vi "Configure Alarm Delay Com.vi"(0 "VISA resource name":refnum<visa-resource-name>, 5 "Comm Channel (001)":string="001", 7 "Alarm Delay Time":cluster{"Hour":i32, "Min":i32, "Sec":i32}={"Hour"=0, "Min"=0, "Sec"=10} {"Sec" min=0 max=59; "Min" min=0 max=59; "Hour" min=0 max=24}, 11 "error in (no error)":errorcluster) -> (4 "VISA resource name out":refnum<visa-resource-name>, 6 "Comm Channel":string, 15 "error out":errorcluster)   [LabVIEW 2020, in "Yokogawa GX Series.lvlib"]
doc: "Sets the alarm delay of a communication channel.\n\nCommand: SAlmDlyCom"
uses:
  <instrlib>/Yokogawa GX Series/Yokogawa GX Series.lvlib
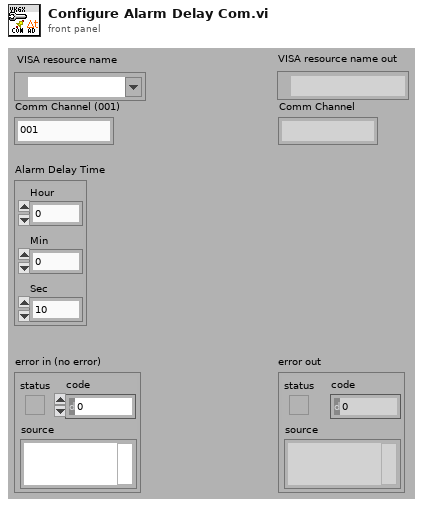
[diagram p1: front panel]
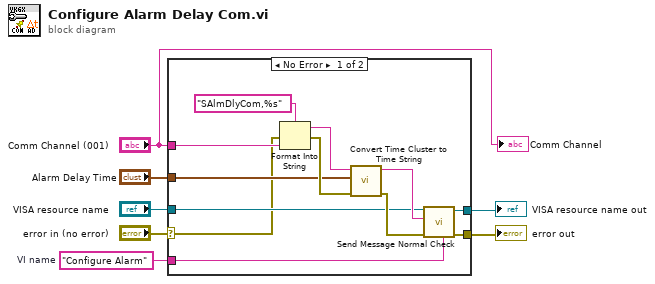
[diagram p0: block diagram]
diagram:
  w3 = "Configure Alarm"  # VI name
  n1 = case shown="No Error" "error in (no error)" {
    selector: "error in (no error)" -> [w8 w20]
    tunnel: [w19 w21] -> w7
    tunnel: "Alarm Delay Time" -> [w13 _]
    tunnel: "VISA resource name" -> [w12 w21]
    tunnel: [w11 w20] -> w4
    tunnel: w3 -> [w10 _]
    tunnel: "Comm Channel (001)" -> [w9 _]
    frame No Error {
      n2 = Format Into String(format string="SAlmDlyCom,%s" ("形式文字列"), error in=w8, w9) -> (resulting string=w17:string, error out=w16:errorcluster)  [unwired: 1 in]
      n3 = call <instrlib>:"Convert Time Cluster to Time String.vi"("error in (no error)"=w16, "Time"=w13, "String"=w17) -> ("error out"=w14:errorcluster, "Time String"=w15:string)  [unwired: 7 in]
      n4 = call <instrlib>:"Send Message Normal Check.vi"("Source (\"\")"=w10, "error in (no error)"=w14, "Send Message (\"\")"=w15, "VISA resource name"=w12) -> ("error out"=w11:errorcluster, "VISA resource name out"=w19:refnum<visa-resource-name>)  [unwired: 2 in, 4 out]
    }
    frame Error {
    }
  }
  "error out" <- w4
  "VISA resource name out" <- w7
  "Comm Channel" <- "Comm Channel (001)"
